vi "CAN TDMS Writer.vi"   [LabVIEW 2014]
uses:
  Global Data.vi
types:
  T1 = enum16{"big-endian, network order", "native, host order", "little-endian"}
  T2 = enum16{"open", "open or create", "create or replace", "create", "open (read-only)"}
  T3 = cluster{"read mode":enum16{"polling", "blocking"}, "write mode":enum16{"polling", "blocking"}}
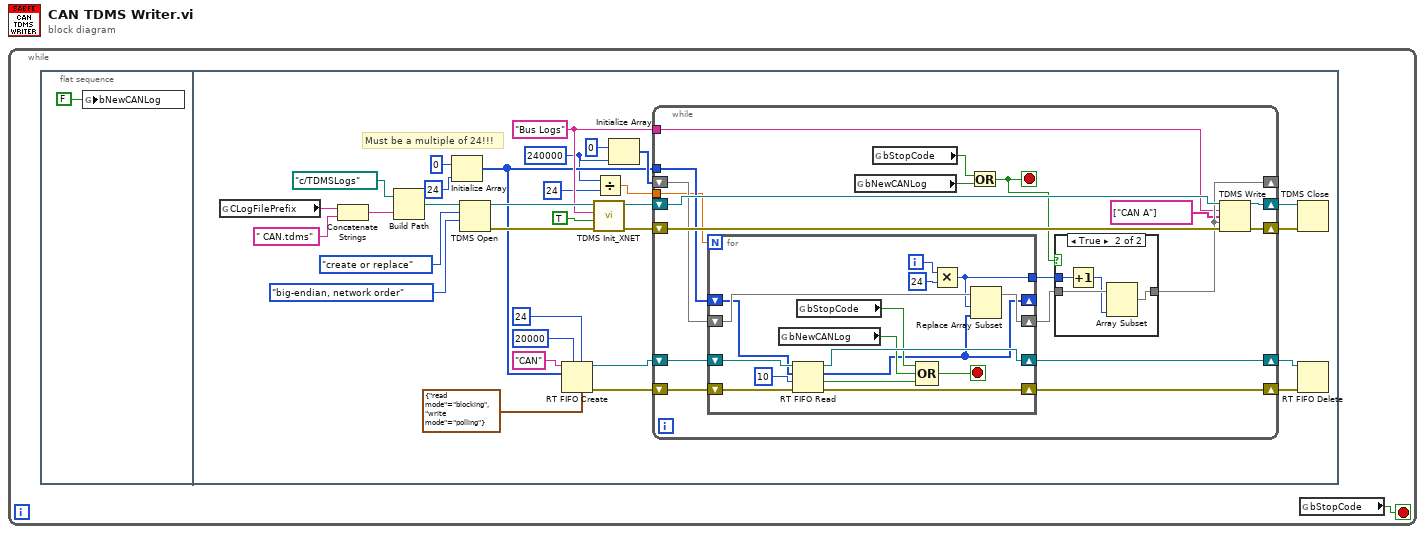
[diagram p0: block diagram]
diagram:
  n1 = while {
    stop <- w1 stop-if-true
    n2 = flat-sequence {
      frame #0 {
        n3 = global write "Global Data.vi" "bNewCANLog"(FALSE ("New MC TDMS")) -> ()
      }
      frame #1 {
        w16 = "Bus Logs" ("group name")
        w5 = 240000 ("dimension size")
        # "Must be a multiple of 24!!!"
        n4 = global read "Global Data.vi" "CLogFilePrefix"() -> (w20:string)
        n5 = Concatenate Strings(w20, " CAN.tdms" ("string")) -> (w19:string)
        n6 = Build Path(base path=path "c:/TDMSLogs", name or relative path=w19) -> (appended path=w23:path)
        n7 = Initialize Array(u8 0 ("element"), 24 ("dimension size")) -> (w9:u8[])
        n8 = TDMS Open(9:T1."big-endian, network order" ("byte order (2:little-endian)"), 10:T2."create or replace" ("operation (0:open)"), 11:w23) -> (0:w15:errorcluster, 3:w17:refnum<k34>)  [unwired: 4 in]
        n9 = RT FIFO Create(0:"CAN" ("name (unnamed)"), 1:w9, 4:u32 20000 ("size (10)"), 6:u32 24 ("elements in array (1)"), 7:T3 {"read mode"=enum."blocking", "write mode"=enum."polling"} ("r/w modes (polling,polling)")) -> (8:w32:refnum<k33>, 11:w31:errorcluster)  [unwired: 3 in, 1 out]
        n10 = call "TDMS Init_XNET.vi"("error in (no error)"=w15, "sbRIO?"=TRUE, "group name"=w16, "tdms file"=w17) -> ("error out"=w14:errorcluster, "tdms file out"=w13:refnum<k34>)  [unwired: 6 in]
        n11 = Divide(x=w5, y=24) -> (x/y=w3:dbl)
        n12 = Initialize Array(u8 0 ("element"), w5) -> (w28:u8[])
        n13 = while {
          shift-right: [w44] -> _
          shift-left: w28 -> [w46]
          shift-right: [w50] -> w25
          shift-left: w32 -> [w52]
          shift-right: [w49] -> w24
          shift-left: w31 -> [w51]
          shift-right: [w38] -> w26
          shift-left: w13 -> [w48]
          shift-right: [w37] -> w27
          shift-left: w14 -> [w47]
          tunnel: w9 -> [w36]
          tunnel: w3 -> [w35]
          tunnel: w16 -> [w34]
          stop <- w40 stop-if-true
          n14 = for {
            N: w35 -> [_]
            shift-right: [w71] -> w50
            shift-left: w52 -> [w73]
            shift-right: [w70] -> w49
            shift-left: w51 -> [w72]
            shift-right: [w67] -> w45
            shift-left: w46 -> [w68]
            tunnel: [w59] -> w43
            shift-right: [w61] -> _
            shift-left: w36 -> [w62]
            i -> [w60]
            stop <- w63 stop-if-true
            n15 = global read "Global Data.vi" "bNewCANLog"() -> (w65:bool)
            n16 = RT FIFO Read(0:w73, 1:w62, 2:10 ("timeout in ms (0)"), 3:w72) -> (8:w71:refnum<k33>, 9:w61:u8[], 10:w64:bool, 11:w70:errorcluster)  [unwired: 1 out]
            n17 = global read "Global Data.vi" "bStopCode"() -> (w66:bool)
            n18 = Compound Arithmetic op=OR(w66, w65, w64) -> (w63:bool)
            n19 = Multiply(x=w60, y=24) -> (x*y=w59:i32)
            n20 = Replace Array Subset(array=w68, new element=w61, index=w59) -> (w67:u8[])
          }
          n21 = global read "Global Data.vi" "bNewCANLog"() -> (w41:bool)
          n22 = global read "Global Data.vi" "bStopCode"() -> (w42:bool)
          n23 = Or(x=w42, y=w41) -> (x .or. y?=w40:bool)
          n24 = case shown="True" w40 {
            tunnel: w45 -> [w53 w57]
            tunnel: [w53 w56] -> w44
            tunnel: w43 -> [_ w54]
            frame False {
            }
            frame True {
              n25 = Increment(x=w54) -> (x+1=w55:i32)
              n26 = Array Subset(array=w57, length=w55) -> (w56:u8[])  [unwired: 1 in]
            }
          }
          n27 = TDMS Write(0:w48, 5:w34, 7:string[] ["CAN A"], 9:w44, 11:w47) -> (4:w38:refnum<k34>, 15:w37:errorcluster)  [unwired: 1 in, 2 out]
        }
        n28 = TDMS Close(8:w27, 11:w26) -> ()  [unwired: 2 out]
        n29 = RT FIFO Delete(0:w25, 3:w24) -> ()  [unwired: 1 in, 1 out]
      }
    }
    n30 = global read "Global Data.vi" "bStopCode"() -> (w1:bool)
  }
